vi "Meters per second to ticks per 100ms (SubVI).vi"(10 "WheelPowerDesired M/S":dbl, 11 "driveCountsPerInch":dbl) -> (3 "Numeric":dbl)   [LabVIEW 2020]
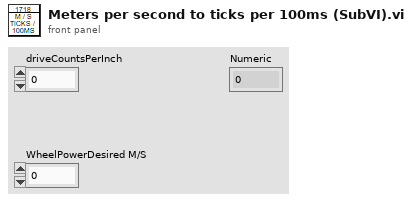
[diagram p1: front panel]
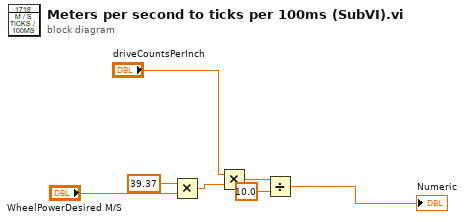
[diagram p0: block diagram]
diagram:
  n1 = Multiply(x=39.37, y="WheelPowerDesired M/S") -> (x*y=w3:dbl)
  n2 = Multiply(x="driveCountsPerInch", y=w3) -> (x*y=w5:dbl)
  n3 = Divide(x=w5, y=10.0) -> (x/y=→"Numeric":dbl)
